vi "Plots listbox popout size.vi"(9 "NumRows":i32, 10 "ItemNames":string[](array[string]), 11 "font":T1) -> (2 "Height":i32, 3 "Text width":i16)   [LabVIEW 2021, in "RocketPlot.lvlib"]
uses:
  RocketPlot.lvlib
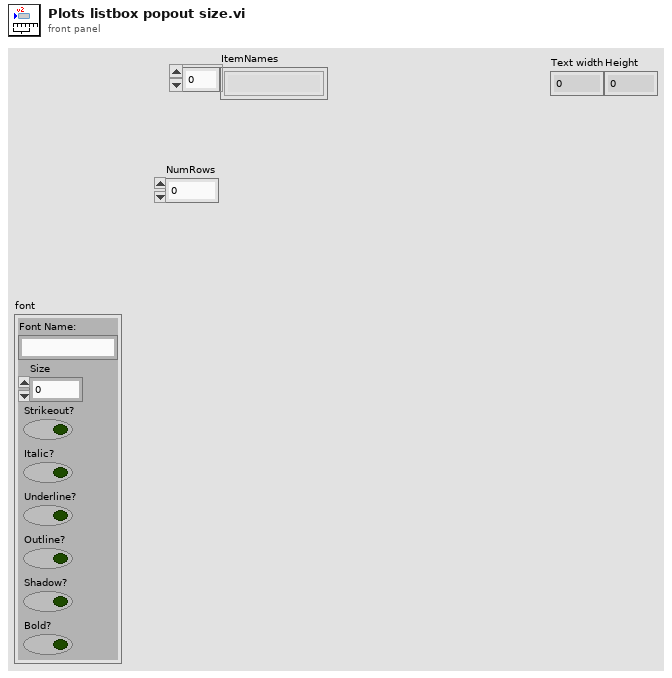
[diagram p1: front panel]
types:
  T1 = cluster{"Font Name:":string, "Size":i16, "Strikeout?":bool, "Italic?":bool, "Underline?":bool, "Outline?":bool, "Shadow?":bool, "Bold?":bool}
  T2 = enum16{"User-specified Font", "Application Font", "System Font", "Dialog Font"}
  T3 = cluster{"left":i16, "top":i16, "right":i16, "bottom":i16}
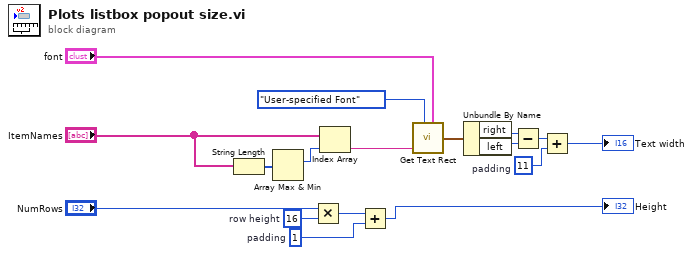
[diagram p0: block diagram]
diagram:
  w1 = 1  # padding
  w3 = 16  # row height
  w12 = i16 11  # padding
  n1 = String Length(string="ItemNames") -> (length=w7:i32[])
  n2 = Array Max & Min(array=w7) -> (max index (indices)=w6:i32)  [unwired: 3 out]
  n3 = Multiply(x="NumRows", y=w3) -> (x*y=w2:i32)
  n4 = Index Array(array="ItemNames", index=w6) -> (element=w5:string)
  n5 = Add(x=w2, y=w1) -> (x+y=→"Height":i32)
  n6 = call <vilib>:"Get Text Rect.vi"("desired font(Application)"=T2."User-specified Font", "text"=w5, "[user-specified font]"="font") -> ("rect"=w8:T3)  [unwired: 6 in]
  n7 = Unbundle By Name(w8) -> ("right"=w9:i16, "left"=w10:i16)
  n8 = Subtract(x=w9, y=w10) -> (x-y=w11:i16)
  n9 = Add(x=w11, y=w12) -> (x+y=→"Text width":i16)
